vi "Reference Rectangle.vi"(8 "error in (no error)":errorcluster, 10 "My VI":string, 11 "Ref VI in":refnum<class "Ref Ctrl.lvclass">) -> (0 "error out":errorcluster, 2 "Rectangle":T1)   [LabVIEW 2019, in "Panel.lvlib" / "Ref Ctrl.lvclass"]
doc: "Returns the center point to use as a reference when positioning the window.\n\n----\nPlease see the following web address for additional documentation and tutorial information:\nhttp://www.mooregoodideas.com/mgi-panel-manager/\n\nAuthor: Derek Trepanier\n\nCopyright (c) 2018, Moore Good Ideas, Inc.\n\nAll rights reserved.\n\nRedistribution and use in source and binary forms, with or without modification, are permitted provided that the following conditions are met:\n\n * Redistributions of source code must retain the above copyright notice, this list of conditions and the following disclaimer.\n * Redistributions in binary form must reproduce the above copyright notice, this list of conditions and the following disclaimer in the documentation and/or other materials provided with the distribution.\n * Neither the name of Moore Good Ideas, Inc. nor the names of its contributors may be used to endorse or promote products derived from this software without specific prior written permission.\n\nTHIS SOFTWARE IS PROVIDED BY THE COPYRIGHT HOLDERS AND CONTRIBUTORS \"AS IS\" AND ANY EXPRESS OR IMPLIED WARRANTIES, INCLUDING, BUT NOT LIMITED TO, THE IMPLIED WARRANTIES OF MERCHANTABILITY AND FITNESS FOR A PARTICULAR PURPOSE ARE DISCLAIMED. IN NO EVENT SHALL THE COPYRIGHT OWNER OR CONTRIBUTORS BE LIABLE FOR ANY DIRECT, INDIRECT, INCIDENTAL, SPECIAL, EXEMPLARY, OR CONSEQUENTIAL DAMAGES (INCLUDING, BUT NOT LIMITED TO, PROCUREMENT OF SUBSTITUTE GOODS OR SERVICES; LOSS OF USE, DATA, OR PROFITS; OR BUSINESS INTERRUPTION) HOWEVER CAUSED AND ON ANY THEORY OF LIABILITY, WHETHER IN CONTRACT, STRICT LIABILITY, OR TORT (INCLUDING NEGLIGENCE OR OTHERWISE) ARISING IN ANY WAY OUT OF THE USE OF THIS SOFTWARE, EVEN IF ADVISED OF THE POSSIBILITY OF SUCH DAMAGE."
uses:
  Ref Ctrl.lvclass
  Ref Ctrl.lvclass/Ref Ctrl.ctl
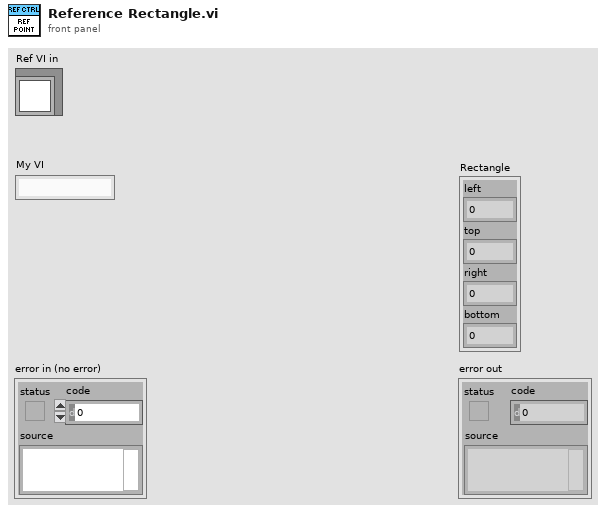
[diagram p1: front panel]
types:
  T1 = cluster{"left":i16, "top":i16, "right":i16, "bottom":i16}
  T2 = typedef "LVPointTypeDef.ctl" = cluster{"Horizontal":i16, "Vertical":i16}
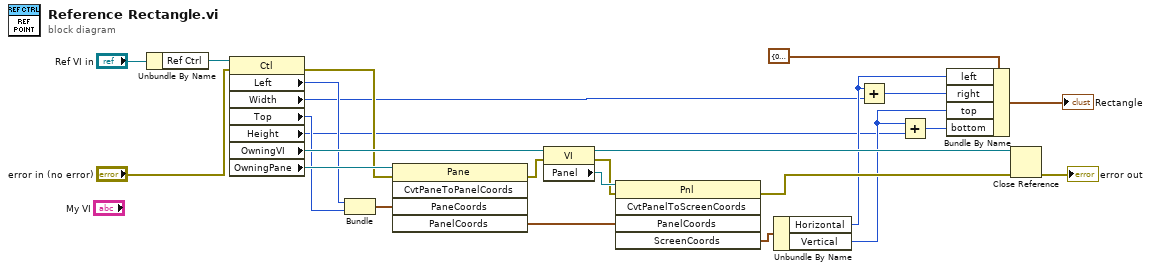
[diagram p0: block diagram]
diagram:
  n1 = Unbundle By Name("Ref VI in") -> ("Ref Ctrl"=w24:refnum<vi>)
  n2 = property class="Ctl"(reference=w24, error in="error in (no error)") -> (error out=w11:errorcluster, "Left"=w15:i32, "Width"=w6:u32, "Top"=w14:i32, "Height"=w2:u32, "OwningVI"=w21:refnum<vi>, "OwningPane"=w22:refnum<vi>)  [unwired: 1 out]
  n3 = Bundle("Left"=w15, "Top"=w14) -> (w13:cluster{"Left":i32, "Top":i32})  [unwired: 1 in]
  n4 = invoke class="Pane" method="CvtPaneToPanelCoords"(reference=w22, error in=w11, "PaneCoords"=w13) -> (error out=w19:errorcluster, "PanelCoords"=w23:T2)  [unwired: 2 in, 3 out]
  n5 = property class="VI"(reference=w21, error in=w19) -> (reference out=w17:refnum<vi>, error out=w18:errorcluster, "Panel"=w20:refnum<vi>)
  n6 = invoke class="Pnl" method="CvtPanelToScreenCoords"(reference=w20, error in=w18, "PanelCoords"=w23) -> (error out=w16:errorcluster, "ScreenCoords"=w8:T2)  [unwired: 2 in, 3 out]
  n7 = Unbundle By Name(w8) -> ("Horizontal"=w7:i16, "Vertical"=w4:i16)
  n8 = Add(x=w7, y=w6) -> (x+y=w5:u32)
  n9 = Add(x=w4, y=w2) -> (x+y=w3:u32)
  n10 = Bundle By Name(cluster=T1 {"left"=0, "top"=0, "right"=0, "bottom"=0} ("Rectangle"), "left"=w7, "right"=w5, "top"=w4, "bottom"=w3) -> (→"Rectangle":T1)
  n11 = Close Reference(reference=w17, error in (no error)=w16) -> (error out=→"error out":errorcluster)
